vi "myRIO_BRig_RT_dataExp_Audio_amp__R.vi"() -> (2 "output_Audio_amp__R":i32)   [LabVIEW 2014]
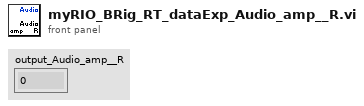
[diagram p1: front panel]
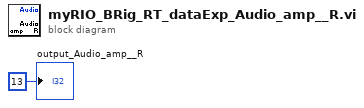
[diagram p0: block diagram]
diagram:
  "output_Audio_amp__R" <- 13 ("output_iBlock")
